vi "TimingTestSelf_Asynchronous.vi"(10 "定时触发自动测试(s)":dbl=1.0, 11 "YTESTER测试数据":T1={"Socket(From1)"=1, "SN"=refnum, "StopFlagRef"=refnum, "YT System Queue"=refnum}) -> ()   [LabVIEW 2017]
uses:
  YtCommon.lvlibp/yt`Step TestData.ctl
  YtCommon.lvlibp/yt`Step System Queue.ctl
  7f9ea692-c834-49a8-aad5-42117919e046.vi
  <vilib>/Utility/error.llb/Clear Errors.vi
  YtCommon.lvlibp/yt`varSystemlib IO Read Variable.vi
  YtCommon.lvlibp
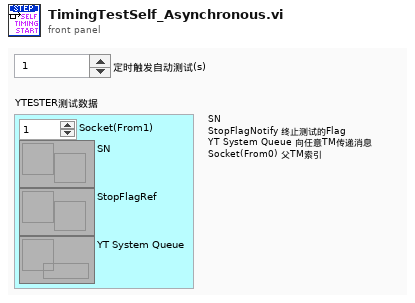
[diagram p1: front panel]
types:
  T1 = typedef "YtCommon.lvlibp/yt`Step TestData.ctl" = cluster{"Socket(From1)":i32, "SN":refnum<notifier>, "StopFlagRef":refnum<notifier>, "YT System Queue":refnum<queue>}
  T2 = typedef "YtCommon.lvlibp/yt`Step System Queue.ctl" = cluster{"Socket(From0)":i32, "Cmd":string, "Data":variant}
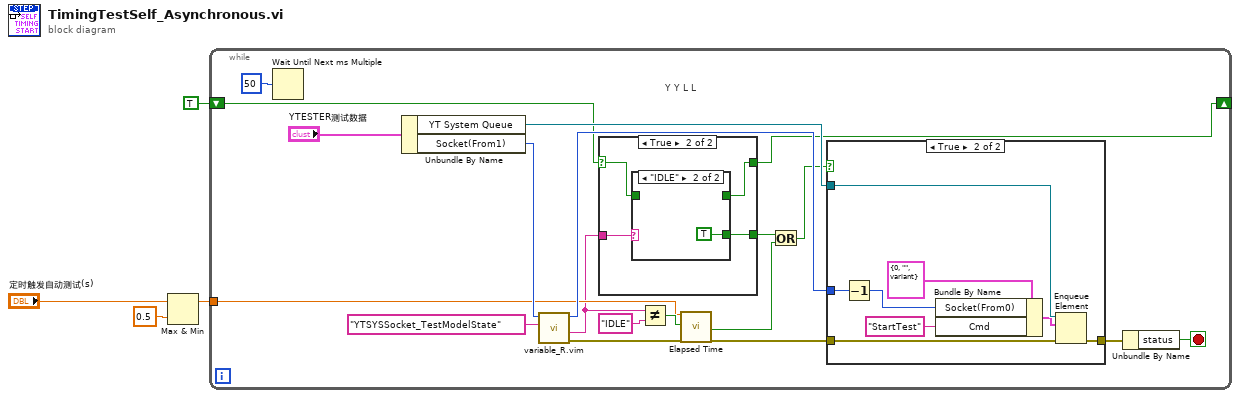
[diagram p0: block diagram]
diagram:
  n1 = Max & Min(x="定时触发自动测试(s)", y=0.5) -> (max(x,y)=w2:dbl)  [unwired: 1 out]
  n2 = while {
    tunnel: w2 -> [w11]
    shift-right: [w7] -> _
    shift-left: TRUE -> [w8]
    stop <- w12 stop-if-true
    # "Y Y L L"
    n3 = Wait Until Next ms Multiple(millisecond multiple=u32 50) -> ()  [unwired: 1 out]
    n4 = Unbundle By Name("YTESTER测试数据") -> ("YT System Queue"=w23:refnum<queue>, "Socket(From1)"=w20:i32)
    n5 = call "variable_R.vim"("待获取变量名称"="YTSYSSocket_TestModelState", "函数池名称"=w20) -> ("error out"=w15:errorcluster, "value"=w6:string, "函数池名称out"=w21:i32)  [unwired: 5 in, 2 out]
    n6 = case shown="True" w8 {
      selector: w8 -> [w24 w26]
      tunnel: [w24 w27] -> w7
      tunnel: w6 -> [_ w28]
      tunnel: [_ w25] -> w5
      frame False {
      }
      frame True {
        n7 = case shown="\"IDLE\"" w28 {
          tunnel: [w29 _] -> w27
          tunnel: w26 -> [w29 _]
          tunnel: [_ TRUE] -> w25
          frame Default {
          }
          frame "IDLE" {
          }
        }
      }
    }
    n8 = Not Equal?(x=w6, y="IDLE") -> (x != y?=w17:bool)
    n9 = call "Elapsed Time"("Time Target (s)"=w11, "Reset"=w17, "error in (no error)"=w15) -> ("Time has Elapsed"=w16:bool, "error out"=w14:errorcluster)  [unwired: 9 in, 6 out]
    n10 = Or(x=w5, y=w16) -> (x .or. y?=w10:bool)
    n11 = case shown="True" w10 {
      tunnel: w23 -> [_ w39]
      tunnel: w21 -> [_ w38]
      tunnel: w14 -> [w31 w33]
      tunnel: [w31 w32] -> w13
      frame False {
      }
      frame True {
        n12 = Decrement(x=w38) -> (x-1=w34:i32)
        n13 = Bundle By Name(cluster=T2 {"Socket(From0)"=0, "Cmd"="", "Data"=variant} ("element"), "Socket(From0)"=w34, "Cmd"="StartTest") -> (w37:T2)
        n14 = Enqueue Element(queue=w39, element=w37, error in (no error)=w33) -> (error out=w32:errorcluster)  [unwired: 1 in, 2 out]
      }
    }
    n15 = Unbundle By Name(w13) -> ("status"=w12:bool)
  }
